vi "Queue IMU Readings.vi"(8 "error in (no error)":errorcluster, 9 "queue":refnum<queue>, 11 "reference":refnum<visa-resource-name>) -> (0 "error out":errorcluster, 1 "queue out":refnum<queue>, 2 "Serial Settings:Number of Bytes at Serial Port":u32, 3 "VISA resource name out":refnum<visa-resource-name>, 5 "timed out?":bool)   [LabVIEW 2012]
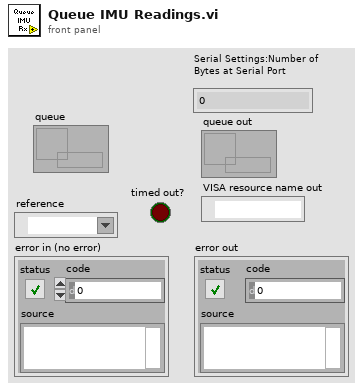
[diagram p1: front panel]
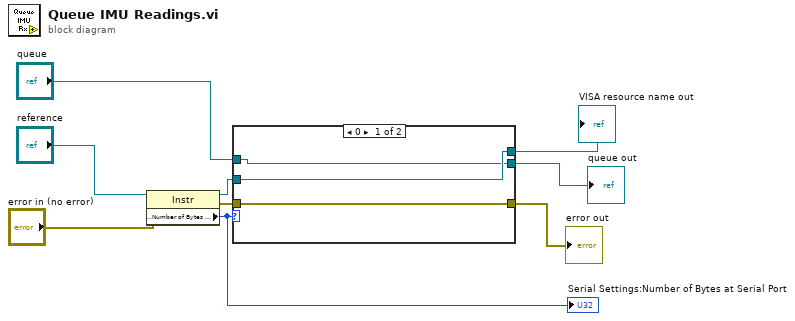
[diagram p0: block diagram]
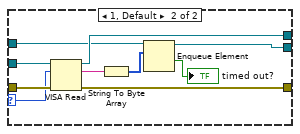
[diagram p2: hidden frame]
diagram:
  n1 = property class="Instr"(reference="reference", error in="error in (no error)") -> (reference out=w9:refnum<visa-resource-name>, error out=w8:errorcluster, "Serial Settings:Number of Bytes at Serial Port"=w7:u32)
  "Serial Settings:Number of Bytes at Serial Port" <- w7
  n2 = case shown="0" w7 {
    selector: w7 -> [_ w14]
    tunnel: w9 -> [w12 w22]
    tunnel: [w12 w21] -> w4
    tunnel: w8 -> [w11 w20]
    tunnel: [w10 w16] -> w5
    tunnel: [w11 w15] -> w6
    tunnel: "queue" -> [w10 w13]
    frame 0 {
    }
    frame 1, Default {
      n3 = VISA Read(VISA resource name=w22, byte count=w14, error in (no error)=w20) -> (VISA resource name out=w21:refnum<visa-resource-name>, read buffer=w19:string, error out=w15:errorcluster)  [unwired: 1 out]
      n4 = String To Byte Array(string=w19) -> (unsigned byte array=w18:u8[])
      n5 = Enqueue Element(queue=w13, element=w18) -> (queue out=w16:refnum<queue>, timed out?=→"timed out?":bool)  [unwired: 2 in, 1 out]
    }
  }
  "error out" <- w6
  "queue out" <- w5
  "VISA resource name out" <- w4
